vi "myRIO_BRig_RT_dataCurrent_laser1_tSel_start.vi"() -> (2 "output_laser1_tSel_start":i32)   [LabVIEW 2014]
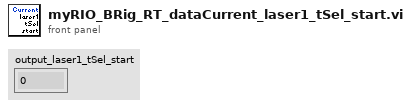
[diagram p1: front panel]
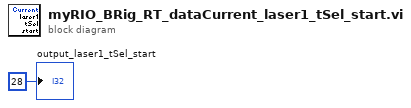
[diagram p0: block diagram]
diagram:
  "output_laser1_tSel_start" <- 28 ("output_iBlock")
